vi "DOperiodic.vi"   [LabVIEW 2015]
doc: "This vi periodically (every 100ms) check the buttons of the joystick. If one button is pressed, the corresponding DO is set to high, the others to false"
types:
  T1 = typedef "WPI_JoystickDevRef.ctl" = cluster{"Device":T2}
  T2 = typedef "WPI_JoystickDeviceEnum.ctl" = enum16{"USB 0", "USB 1", "USB 2", "USB 3", "USB 4", "USB 5"}
  T3 = typedef "DOs.ctl" = cluster{"DIOChannel":T4, "Name":string}[]
  T4 = typedef "FPGA_DIOChannel.ctl" = enum8{"DIO 1", "DIO 2", "DIO 3", "DIO 4", "DIO 5", "DIO 6", "DIO 7", "DIO 8", "DIO 9", "DIO 10", "DIO 11", "DIO 12", "DIO 13", "DIO 14", "Invalid"}
  T5 = typedef "WPI_DigitalOutputDevRef.ctl" = cluster{"Digital Module":T6, "DIO Channel":T4, "DevStatus":errorcluster}
  T6 = typedef "FPGA_TypedefDigitalModule.ctl" = enum16{"Digital Module 1", "Digital Module 2"}
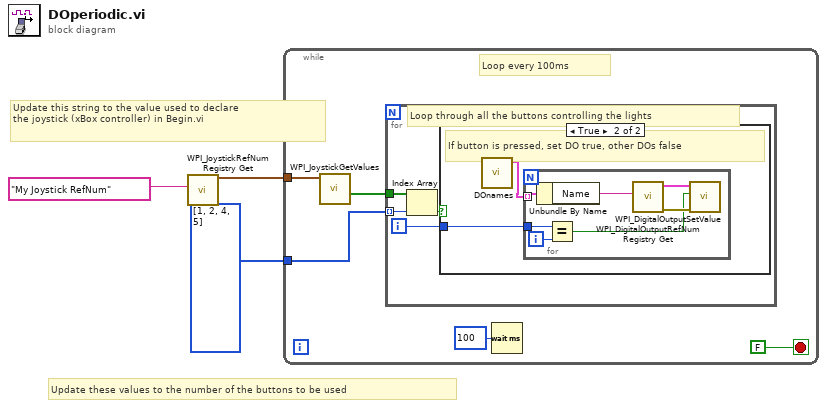
[diagram p0: block diagram]
diagram:
  # "Update these values to the number of the buttons to be used"
  # "Update this string to the value used to declare \nthe joystick (xBox controller) in Begin.vi"
  n1 = call <vilib>:"WPI_JoystickRefNum Registry Get.vi"("refnum name"="My Joystick RefNum") -> ("JoystickDevRef"=w2:T1)  [unwired: 9 in, 1 out]
  n2 = while {
    tunnel: w2 -> [w6]
    tunnel: i32[] [1, 2, 4, 5] ("index") -> [w4]
    stop <- FALSE stop-if-true
    # "Loop every 100ms"
    n3 = call <vilib>:"WPI_JoystickGetValues.vi"("JoystickDevRef"=w6) -> ("Buttons"=w5:bool[])  [unwired: 6 in, 4 out]
    n4 = for {
      tunnel: w5 -> [w12]
      tunnel: w4 -> [w11] mode=indexing
      i -> [w9]
      # "Loop through all the buttons controlling the lights"
      n5 = Index Array(array=w12, index=w11) -> (element=w10:bool)
      n6 = case shown="True" w10 {
        tunnel: w9 -> [_ w13]
        frame False {
          # "If button is not pressed, do nothing"
        }
        frame True {
          # "If button is pressed, set DO true, other DOs false"
          n7 = call "DOnames.vi"() -> ("DIO Channel"=w14:T3)  [unwired: 11 in]
          n8 = for {
            tunnel: w14 -> [w19] mode=indexing
            tunnel: w13 -> [w16]
            i -> [w17]
            n9 = Unbundle By Name(w19) -> ("Name"=w18:string)
            n10 = Equal?(x=w16, y=w17) -> (x = y?=w15:bool)
            n11 = call <vilib>:"WPI_DigitalOutputRefNum Registry Get.vi"("refnum name"=w18) -> ("error out"=w21:errorcluster, "DigitalOutputDevRef"=w20:T5)  [unwired: 9 in]
            n12 = call <vilib>:"WPI_DigitalOutputSetValue.vi"("error in (no error)"=w21, "Value"=w15, "DigitalOutputDevRef"=w20) -> ()  [unwired: 7 in, 2 out]
          }
        }
      }
    }
    n13 = Wait (ms)(milliseconds to wait=u32 100) -> ()  [unwired: 1 out]
  }
